vi "ief_get_system_parameter_min.vi"(3 "error in (no error)":errorcluster, 4 "System Parameter":u16(ring) items=["language", "number of axes", "start entry number", "stop entry number", "manual release entry number", "standby entry number", "malfunction output number", "autostart", "not in use", "not in use", "not in use", "not in use", "not in use", "not in use", "activate teleservice entry number", "activate teleservice output number", "profibus DP adress", "not in use", "profibus diagnosis active", "basic operation state of PA control"], 5 "Tagprefix in":refnum<k21>) -> (0 "error out (no error)":errorcluster, 1 "Minimum Parameter Value":i32, 2 "Tagprefix out":refnum<k21>)   [LabVIEW 2015, in "IEF Werner.lvlib"]
doc: "The VI returns the present minimum value of the chosen system parameter.\n\nSystem Parameter Range:\n01 hex, 1 dec - language\n02 hex, 2 dec - number of axes\n03 hex, 3 dec - start enty number\n04 hex, 4 dec - stop entry number\n05 hex, 5 dec - manual release entry number\n06 hex, 6 dec - standby entry number \n07 hex, 7 dec - error output number\n08 hex, 8 dec - autostart\n0F hex, 15 dec - activate teleservice entry number\n10 hex, 16 dec - activate teleservice output number\n11 hex, 17 dec - profibus DP adress\n13 hex, 19 dec - profibus diagnosis active \n14 hex, 20 dec - basic operation state of PA control"
uses:
  IEF Werner.lvlib
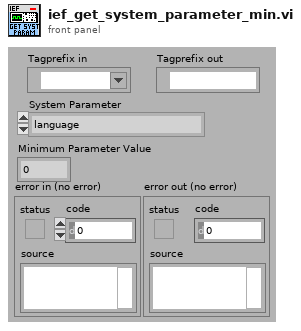
[diagram p1: front panel]
types:
  T1 = typedef "Semaphore RefNum" = refnum<k1>
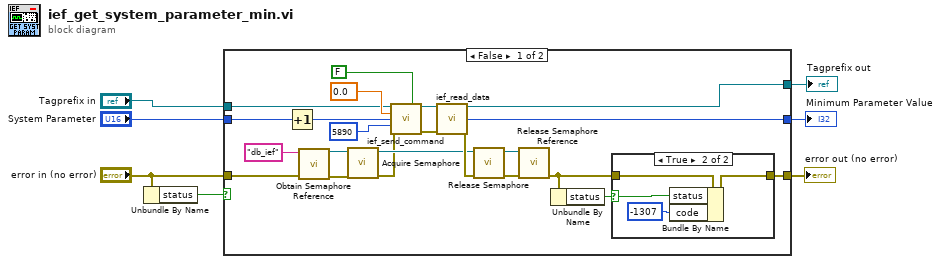
[diagram p0: block diagram]
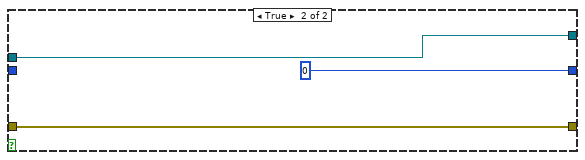
[diagram p3: hidden frame]
diagram:
  n1 = Unbundle By Name("error in (no error)") -> ("status"=w6:bool)
  n2 = case shown="False" w6 {
    tunnel: "error in (no error)" -> [w12 w37]
    tunnel: "System Parameter" -> [w25 _]
    tunnel: [w27 w37] -> w4
    tunnel: [w11 u32 0 ("value uint 32")] -> w3
    tunnel: "Tagprefix in" -> [w10 w36]
    tunnel: [w8 w36] -> w1
    frame False {
      n3 = Increment(x=w25) -> (x+1=w23:u16)
      n4 = call <vilib>:"Obtain Semaphore Reference.vi"("error in (no error)"=w12, "name (unnamed)"="db_ief") -> ("error out"=w17:errorcluster, "semaphore"=w16:T1)  [unwired: 3 in, 1 out]
      n5 = call <vilib>:"Acquire Semaphore.vi"("error in (no error)"=w17, "semaphore"=w16) -> ("error out"=w13:errorcluster, "semaphore out"=w18:T1)  [unwired: 3 in, 1 out]
      n6 = call "ief_send_command.vi"("Tagprefix in"=w10, "Command datum of type real"=FALSE, "Command datum"=sgl 0.0, "Command parameter"=w23, "Command code"=u16 5890, "error in (no error)"=w13) -> ("Tagprefix out"=w9:refnum<k21>, "error out (no error)"=w28:errorcluster)  [unwired: 4 in, 4 out]
      n7 = call "ief_read_data.vi"("Tagprefix in"=w9, "error in (no error)"=w28) -> ("Tagprefix out"=w8:refnum<k21>, "value uint 32"=w11:u32, "error out (no error)"=w26:errorcluster)  [unwired: 7 in, 4 out]
      n8 = call <vilib>:"Release Semaphore.vi"("error in (no error)"=w26, "semaphore"=w18) -> ("error out"=w19:errorcluster, "semaphore out"=w20:T1)  [unwired: 4 in]
      n9 = call <vilib>:"Release Semaphore Reference.vi"("error in (no error)"=w19, "semaphore"=w20) -> ("error out"=w14:errorcluster)  [unwired: 8 in, 1 out]
      n10 = Unbundle By Name(w14) -> ("status"=w21:bool)
      n11 = case shown="True" w21 {
        selector: w21 -> [_ w32]
        tunnel: w14 -> [w30 w34]
        tunnel: [w30 w33] -> w27
        frame False {
        }
        frame True {
          n12 = Bundle By Name(cluster=w34, "status"=w32, "code"=-1307) -> (w33:errorcluster)
        }
      }
    }
    frame True {
    }
  }
  "error out (no error)" <- w4
  "Minimum Parameter Value" <- w3
  "Tagprefix out" <- w1
